vi "Fetch Measurement (Multiple).vi"(8 "error in (no error)":errorcluster, 10 "Timeout (10000 ms)":u32=10000, 11 "VISA resource name":refnum<visa-resource-name>) -> (0 "error out":errorcluster, 2 "Measurements":dbl[](array[numeric]), 3 "VISA resource name out":refnum<visa-resource-name>)   [LabVIEW 2024, in "Agilent 532XX Series.lvlib"]
doc: "Queries and retrieves multiple measurement results.\n\n<B>Note:</B> This VI does not check the instrument status. Typically, you call this VI only in a sequence of calls to other low-level instrument driver VIs. The sequence performs one operation. You use the low-level VIs to optimize one or more aspects of interaction with the instrument."
uses:
  Agilent 532XX Series.lvlib
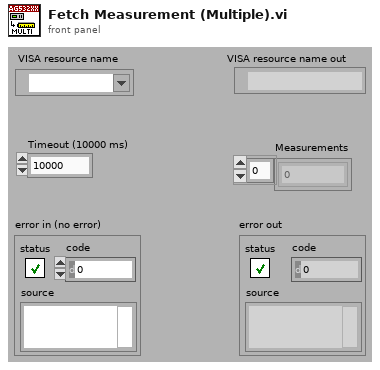
[diagram p1: front panel]
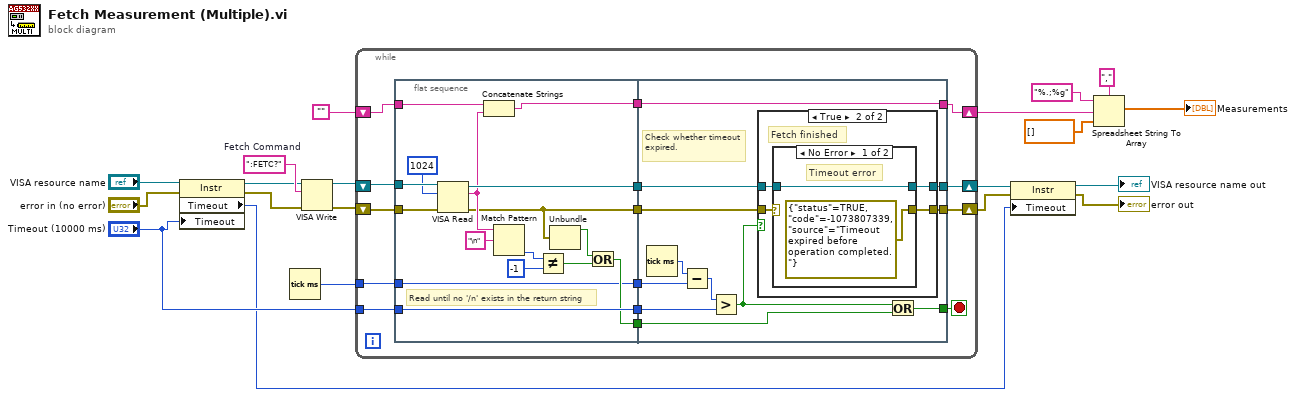
[diagram p0: block diagram]
diagram:
  w18 = ":FETC?"  # Fetch Command
  n1 = property class="Instr"(reference="VISA resource name", error in="error in (no error)", "Timeout"="Timeout (10000 ms)") -> (reference out=w14:refnum<visa-resource-name>, error out=w15:errorcluster, "Timeout"=w10:u32)
  n2 = Tick Count (ms)() -> (millisecond timer value=w12:u32)
  n3 = VISA Write(VISA resource name=w14, write buffer=w18, error in (no error)=w15) -> (VISA resource name out=w2:refnum<visa-resource-name>, error out=w1:errorcluster)  [unwired: 1 out]
  n4 = while {
    shift-right: [w31] -> w3
    shift-left: "" -> [w32]
    tunnel: w12 -> [w25]
    tunnel: "Timeout (10000 ms)" -> [w24]
    shift-right: [w34] -> w9
    shift-left: w2 -> [w33]
    shift-right: [w30] -> w8
    shift-left: w1 -> [w35]
    stop <- w21 stop-if-true
    n5 = flat-sequence {
      tunnel: w35 -> [w51]
      tunnel: w33 -> [w49]
      tunnel: w32 -> [w47]
      tunnel: [w50] -> w29
      tunnel: [w46] -> w28
      tunnel: [w41] -> w27
      tunnel: [w36] -> w26
      tunnel: w25 -> [w36]
      tunnel: w24 -> [w39]
      tunnel: [w39] -> w23
      tunnel: [w37] -> w22
      tunnel: [w58] -> w30
      tunnel: [w63] -> w31
      tunnel: [w55] -> w34
      tunnel: w29 -> [w56]
      tunnel: w28 -> [w63]
      tunnel: w27 -> [w57]
      tunnel: w26 -> [w61]
      tunnel: w23 -> [w59]
      tunnel: w22 -> [w54]
      tunnel: [w52] -> w21
      frame #0 {
        # "Read until no '/n' exists in the return string"
        n6 = VISA Read(VISA resource name=w49, byte count=u32 1024, error in (no error)=w51) -> (VISA resource name out=w50:refnum<visa-resource-name>, read buffer=w45:string, error out=w41:errorcluster)  [unwired: 1 out]
        n7 = Concatenate Strings(w47, w45) -> (w46:string)
        n8 = Match Pattern(string=w45, regular expression="\n") -> (offset past match=w44:i32)  [unwired: 4 out]
        n9 = Not Equal?(x=w44, y=-1) -> (x != y?=w40:bool)
        n10 = Unbundle(w41) -> ("status"=w38:bool)  [unwired: 2 out]
        n11 = Or(x=w38, y=w40) -> (x .or. y?=w37:bool)
      }
      frame #1 {
        # "Check whether timeout\nexpired."
        n12 = Tick Count (ms)() -> (millisecond timer value=w62:u32)
        n13 = Subtract(x=w62, y=w61) -> (x-y=w60:u32)
        n14 = Greater?(x=w60, y=w59) -> (0:w53:bool)
        n15 = case shown="True" w53 {
          tunnel: [w65 w69] -> w58
          tunnel: w57 -> [w65 w66]
          tunnel: w56 -> [w64 w68]
          tunnel: [w64 w67] -> w55
          frame False {
            # "continue fetch"
          }
          frame True {
            # "Fetch finished"
            n16 = case shown="No Error" w66 {
              selector: w66 -> [_ w72]
              tunnel: [errorcluster {"status"=TRUE, "code"=-1073807339, "source"="Timeout expired before operation completed."} ("error out") w72] -> w69
              tunnel: w68 -> [w70 w73]
              tunnel: [w70 w73] -> w67
              frame No Error {
                # "Timeout error"
              }
              frame Error {
              }
            }
          }
        }
        n17 = Or(x=w53, y=w54) -> (x .or. y?=w52:bool)
      }
    }
  }
  n18 = property class="Instr"(reference=w9, error in=w8, "Timeout"=w10) -> (reference out=→"VISA resource name out":refnum<visa-resource-name>, error out=→"error out":errorcluster)
  n19 = Spreadsheet String To Array(delimiter (Tab)=",", format string="%.;%g", spreadsheet string=w3, array type (2D Dbl)=dbl[] [] ("Results")) -> (array=→"Measurements":dbl[])
